vi "SSL Detection Frame Robots Kalman Estimator.vi"(5 "Time Stamp":timestamp, 7 "Life Time":dbl=1.0, 11 "Robots":T1[](array[typedef]) {"height" format="%+4.3f"; "pixel_y" format="%+4.3f"; "pixel_x" format="%+4.3f"; "orientation" format="%+4.3f"; "y" format="%+4.3f"; "confidence" format="%4.3f"; "x" format="%+4.3f"}) -> (3 "Robots Out":T1[](array[typedef]) {"height" format="%+4.3f"; "pixel_y" format="%+4.3f"; "pixel_x" format="%+4.3f"; "orientation" format="%+4.3f"; "y" format="%+4.3f"; "confidence" format="%4.3f"; "x" format="%+4.3f"})   [LabVIEW 2016]
uses:
  SSL Detection Robot.ctl
  <vilib>/Analysis/Matrix/Datatypes/RealMatrix.ctl
  <vilib>/Analysis/_algsub.llb/Real Vector Norm.vi
  <vilib>/Analysis/Matrix/Numeric/Conversions/Array To Matrix - RA.vi
  <vilib>/Analysis/Matrix/Numeric/Subtract/Subtract - RM,RM.vi
  <vilib>/Analysis/NI_AALPro.lvlib
  <vilib>/Analysis/Matrix/NI_Matrix.lvlib
panel:
  in  "Robots Out 2":T3(array[cluster]) {"Detection Robot"."height" format="%+4.3f"; "Detection Robot"."pixel_y" format="%+4.3f"; "Detection Robot"."pixel_x" format="%+4.3f"; "Detection Robot"."orientation" format="%+4.3f"; "Detection Robot"."y" format="%+4.3f"; "Detection Robot"."confidence" format="%4.3f"; "Detection Robot"."x" format="%+4.3f"}
  out "A-B":dbl[][](array[numeric])
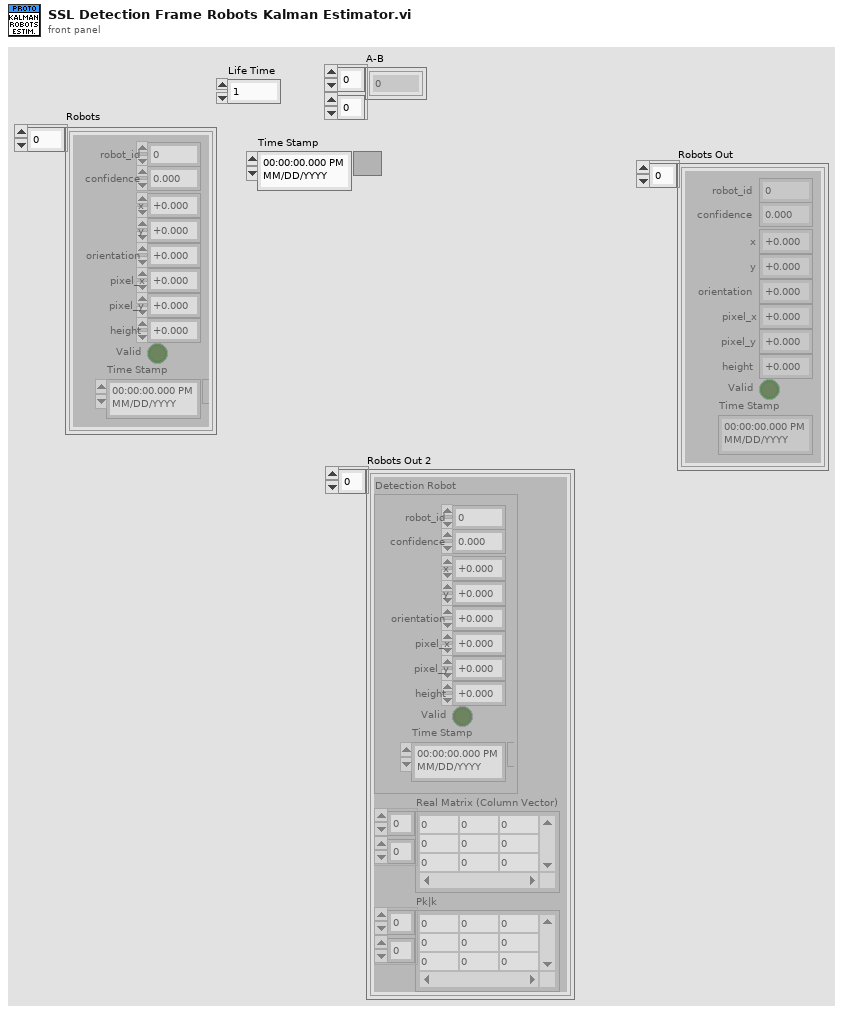
[diagram p1: front panel]
types:
  T1 = typedef "SSL Detection Robot.ctl" = cluster{"x":sgl, "robot_id":u32, "confidence":sgl, "y":sgl, "orientation":sgl, "pixel_x":sgl, "pixel_y":sgl, "height":sgl, "Valid":bool, "Time Stamp":timestamp}
  T2 = typedef "NI_Matrix.lvlib/RealMatrix.ctl" = dbl[][]
  T3 = cluster{"Detection Robot":T1, "Real Matrix (Column Vector)":T2, "Pk|k":T2}[]
  T4 = cluster{"Detection Robot":T1, "Real Matrix (Column Vector)":T2, "Pk|k":T2}
  T5 = cluster{"Detection Robot out":T1, "x_k|k":T2, "Pk|k":T2}
  T6 = cluster{"Detection Robot":T1, "Real Matrix (Column Vector)":T2, dbl[][]}
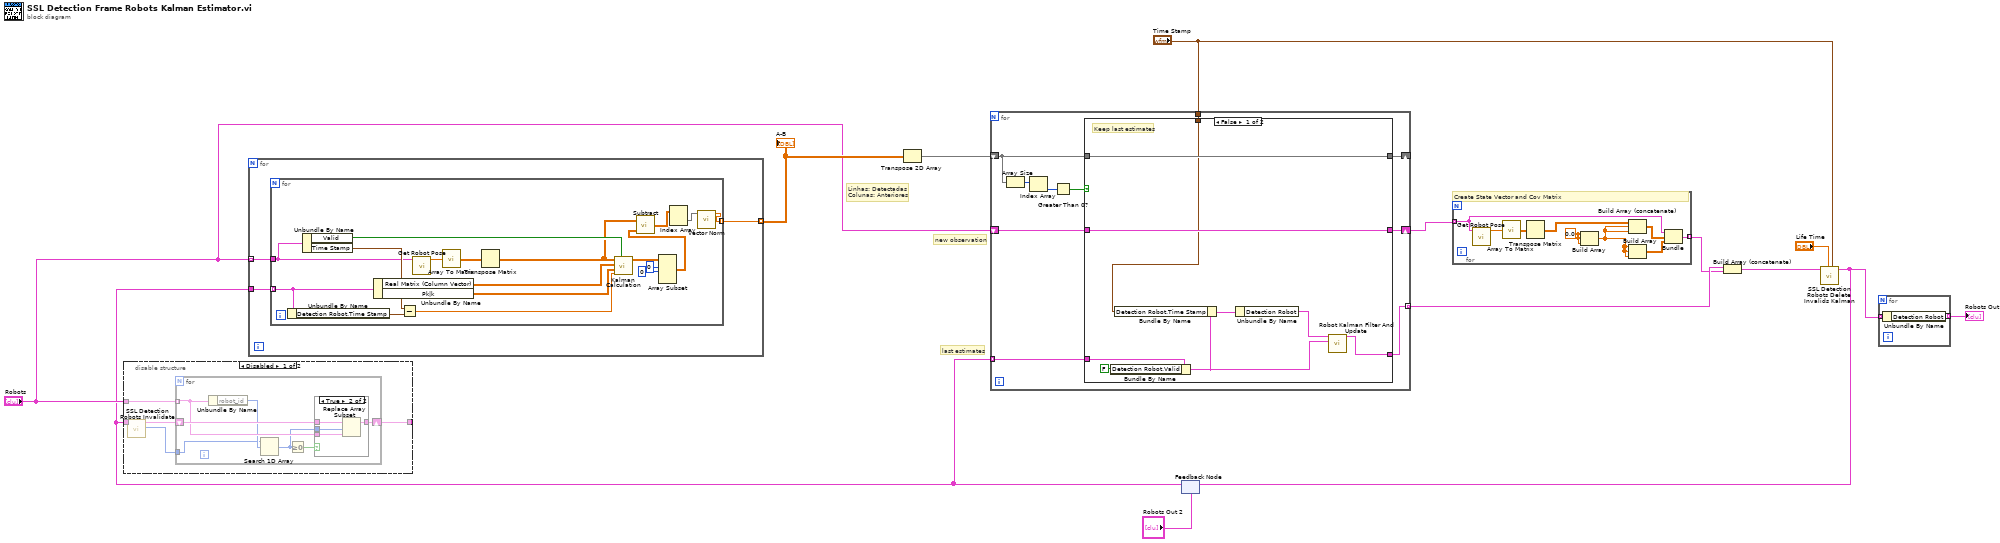
[diagram p0: block diagram]
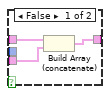
[diagram p2: hidden frame]
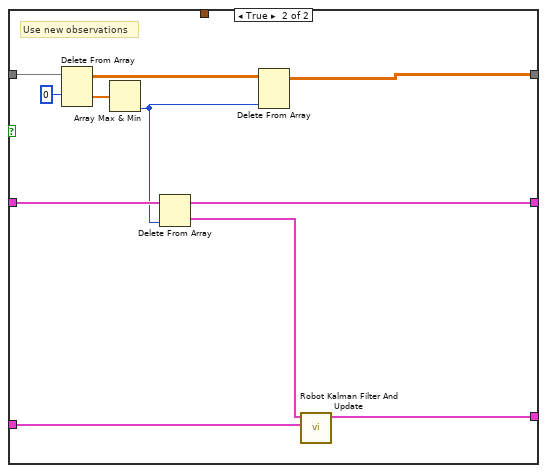
[diagram p4: hidden frame]
diagram:
  # "Linhas: Detectadas\nColunas: Anteriores"
  # "last estimates"
  # "new observation"
  n1 = feedback #1("Robots Out 2") -> (w2:T3)
  n2 = disable-structure shown="Disabled" {
    disable-tunnel: [w17 _] -> _
    disable-tunnel: "Robots" -> [w15 _]
    disable-tunnel: w2 -> [w14 _]
    frame Disabled {
      n3 = call "SSL Detection Robots Invalidate.vi"("Robots"=w14) -> ("Indexes"=w16:u32[], "Robots Invalidated"=w18:T1[])  [unwired: 9 in]
      n4 = for {
        tunnel: w15 -> [w23] mode=indexing
        shift-right: [w24] -> w17
        shift-left: w18 -> [w25]
        tunnel: w16 -> [w21]
        n5 = Unbundle By Name(w23) -> ("robot_id"=w22:u32)
        n6 = Search 1D Array(1D array=w21, element=w22) -> (index of element=w19:i32)  [unwired: 1 in]
        n7 = Greater Or Equal To 0?(x=w19) -> (x >= 0?=w20:bool)
        n8 = case shown="True" w20 {
          tunnel: w25 -> [w27 w32]
          tunnel: [w26 w31] -> w24
          tunnel: w23 -> [w28 w30]
          tunnel: w19 -> [_ w29]
          frame False {
            n9 = Build Array (concatenate)(w27, w28) -> (w26:T1[])
          }
          frame True {
            n10 = Replace Array Subset(array=w32, new element=w30, index=w29) -> (w31:T1[])
          }
        }
      }
    }
    frame Enabled {
    }
  }
  n11 = for {
    tunnel: w2 -> [w35]
    tunnel: "Robots" -> [w34] mode=indexing
    tunnel: [w33] -> w10 mode=indexing
    n12 = for {
      tunnel: w35 -> [w36] mode=indexing
      tunnel: w34 -> [w40]
      tunnel: [w48] -> w33 mode=indexing
      n13 = Unbundle By Name(w36) -> ("Detection Robot.Time Stamp"=w43:timestamp)
      n14 = Unbundle By Name(w40) -> ("Valid"=w53:bool, "Time Stamp"=w42:timestamp)
      n15 = Unbundle By Name(w36) -> ("Real Matrix (Column Vector)"=w45:T2, "Pk|k"=w44:T2)
      n16 = Subtract(x=w42, y=w43) -> (x-y=w41:dbl)
      n17 = call "Get Robot Pose.vi"("Detection Robot"=w40) -> ("Pose"=w38:sgl[])  [unwired: 10 in]
      n18 = call-poly <vilib>:"Array To Matrix.vi"("Real 1D Array"=w38) -> ("Real Matrix (Column Vector)"=w39:T2)
      n19 = Transpose Matrix(1:w39) -> (0:w37:T2)
      n20 = call "Kalman Calculation.vi"("Use Observation"=w53, "iteração"=w41, "Pk-1|k-1"=w44, "x_k-1|k-1"=w45, "z_k"=w37) -> ("x_k|k"=w51:T2)  [unwired: 4 in, 2 out]
      n21 = Array Subset(array=w51, index (row)=0 ("row 1"), length (row)=0 ("row N")) -> (w52:T2)  [unwired: 2 in]
      n22 = call-poly <vilib>:"Subtract.vi"("Real Matrix B"=w52, "Real Matrix A"=w37) -> ("A - B"=w47:T2)
      n23 = Index Array(array=w47) -> (element=w46:dbl[])  [unwired: 2 in]
      n24 = call-poly <vilib>:"Vector Norm.vi"("Input Vector"=w46) -> ("norm"=w48:dbl)  [unwired: 9 in, 1 out]
    }
  }
  "A-B" <- w10
  n25 = Transpose 2D Array(2D array=w10) -> (transposed array=w11:dbl[][])
  n26 = for {
    shift-right: [w62] -> _
    shift-left: w11 -> [w58]
    shift-right: [w61] -> w8
    shift-left: "Robots" -> [w63]
    tunnel: [w60] -> w7 mode=indexing
    tunnel: w2 -> [w59] mode=indexing
    tunnel: "Time Stamp" -> [w54]
    n27 = Array Size(array=w58) -> (size(s)=w56:i32[])
    n28 = Index Array(array=w56) -> (element=w55:i32)  [unwired: 1 in]
    n29 = Greater Than 0?(x=w55) -> (x > 0?=w57:bool)
    n30 = case shown="False" w57 {
      tunnel: w58 -> [w72 w83]
      tunnel: w63 -> [w71 w80]
      tunnel: [w72 w78] -> w62
      tunnel: [w71 w76] -> w61
      tunnel: [w67 w75] -> w60
      tunnel: w59 -> [w66 w73]
      tunnel: w54 -> [w69 _]
      frame False {
        # "Keep last estimates"
        n31 = Bundle By Name(cluster=w66, "Detection Robot.Valid"=FALSE ("Detection Ball.Valid")) -> (w64:T4)
        n32 = Bundle By Name(cluster=w64, "Detection Robot.Time Stamp"=w69) -> (w68:T4)
        n33 = Unbundle By Name(w68) -> ("Detection Robot"=w65:T1)
        n34 = call "Robot Kalman Filter And Update.vi"("Cluster in"=w64, "Detection Robot"=w65) -> ("Cluster out"=w67:T5)  [unwired: 9 in]
      }
      frame True {
        # "Use new observations"
        n35 = Delete From Array(array=w83, index (row)=0) -> (deleted portion=w81:dbl[], array with subset deleted=w79:dbl[][])  [unwired: 2 in]
        n36 = Array Max & Min(array=w81) -> (min index (indices)=w77:i32)  [unwired: 3 out]
        n37 = Delete From Array(array=w80, index=w77) -> (deleted portion=w74:T1, array with subset deleted=w76:T1[])  [unwired: 1 in]
        n38 = Delete From Array(array=w79, index (col)=w77) -> (array with subset deleted=w78:dbl[][])  [unwired: 2 in, 1 out]
        n39 = call "Robot Kalman Filter And Update.vi"("Cluster in"=w73, "Detection Robot"=w74) -> ("Cluster out"=w75:T5)  [unwired: 9 in]
      }
    }
  }
  n40 = for {
    tunnel: w8 -> [w85] mode=indexing
    tunnel: [w88] -> w6 mode=indexing
    w92 = 0.0 ("element")
    # "Create State Vector and Cov Matrix"
    n41 = call "Get Robot Pose.vi"("Detection Robot"=w85) -> ("Pose"=w87:sgl[])  [unwired: 10 in]
    n42 = call-poly <vilib>:"Array To Matrix.vi"("Real 1D Array"=w87) -> ("Real Matrix (Column Vector)"=w86:T2)
    n43 = Transpose Matrix(1:w86) -> (0:w84:T2)
    n44 = Build Array(w92, w92, w92) -> (w91:dbl[])
    n45 = Build Array(w91, w91, w91) -> (w90:dbl[][])
    n46 = Build Array (concatenate)(w84, w91, w91) -> (w89:T2)
    n47 = Bundle("Detection Robot"=w85, "Real Matrix (Column Vector)"=w89, w90) -> (w88:T6)  [unwired: 1 in]
  }
  n48 = Build Array (concatenate)(w7, w6) -> (w1:T3)
  n49 = call "SSL Detection Robots Delete Invalids Kalman.vi"("Now"="Time Stamp", "Life Time"="Life Time", "Robots In"=w1) -> ("Robots Out"=w4:T3)  [unwired: 8 in]
  n50 = feedback-in #1(w4) -> ()
  n51 = for {
    tunnel: w4 -> [w94] mode=indexing
    tunnel: [w93] -> w5 mode=indexing
    n52 = Unbundle By Name(w94) -> ("Detection Robot"=w93:T1)
  }
  "Robots Out" <- w5
